vi "Push to startup and reboot machine.vi"(9 "Password":string="labview===", 10 "username":string="lvadmin", 11 "Array":string[](array[string])) -> ()   [LabVIEW 2013]
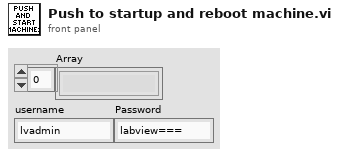
[diagram p1: front panel]
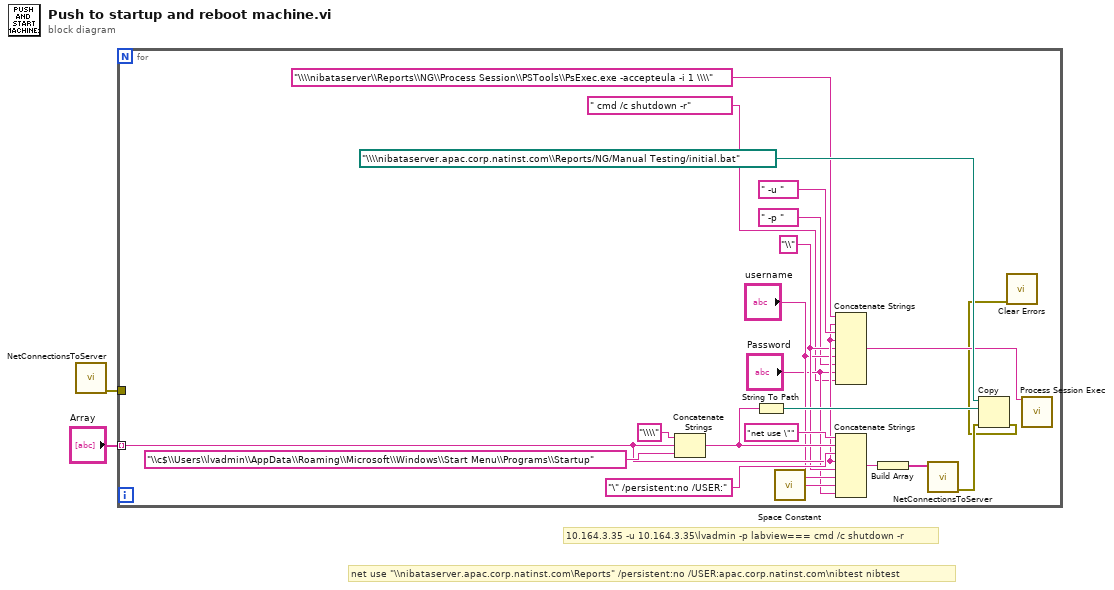
[diagram p0: block diagram]
diagram:
  # "net use \"\\\\nibataserver.apac.corp.natinst.com\\Reports\" /persistent:no /USER:apac.corp.natinst.com\\nibtest nibtest"
  # "10.164.3.35 -u 10.164.3.35\\lvadmin -p labview=== cmd /c shutdown -r"
  n1 = call "NetConnectionsToServer.vi"() -> ("error out"=w1:errorcluster)  [unwired: 11 in]
  n2 = for {
    tunnel: "Array" -> [w10] mode=indexing
    tunnel: w1 -> [_]
    w9 = "\\"
    n3 = Concatenate Strings("\\\\" ("string"), w10, "\\c$\\Users\\lvadmin\\AppData\\Roaming\\Microsoft\\Windows\\Start Menu\\Programs\\Startup" ("string")) -> (w15:string)
    n4 = String To Path(string=w15) -> (path=w14:path)
    n5 = call <vilib>:"Space Constant.vi"() -> ("String"=w13:string)
    n6 = Concatenate Strings("\\\\nibataserver\\Reports\\NG\\Process Session\\PSTools\\PsExec.exe -accepteula -i 1 \\\\" ("command line"), w10, " -u " ("string"), w10, w9, "username", " -p " ("string"), "Password", " cmd /c shutdown -r" ("string")) -> (w4:string)
    n7 = Concatenate Strings("net use \"" ("string"), w15, "\" /persistent:no /USER:" ("string"), w10, w9, "username", w13, "Password") -> (w18:string)
    n8 = Build Array(w18) -> (w17:string[])
    n9 = call "NetConnectionsToServer.vi"("Array"=w17) -> ("error out"=w16:errorcluster)  [unwired: 10 in]
    n10 = Copy(8:w16, 10:w14, 11:path "\\\\nibataserver.apac.corp.natinst.com\\Reports/NG/Manual Testing/initial.bat" ("source path")) -> (0:w3:errorcluster)  [unwired: 2 in, 2 out]
    n11 = call <vilib>:"Clear Errors.vi"("error in (no error)"=w3) -> ()  [unwired: 6 in, 1 out]
    n12 = call "Process Session Exec.vi"("command line"=w4) -> ()  [unwired: 10 in, 5 out]
  }
